vi "Get Selection from TreeBrowserWF.vi"(8 "error in (no error)":errorcluster, 10 "Input Channels":variant, 11 ".NET Refnum in":refnum<k24>) -> (0 "error out":errorcluster, 3 "Input Channel Selections":T1[](array[typedef]))   [LabVIEW 2019, in "Protection and Counter Support System Explorer.lvlib"]
uses:
  Protection and Counter Support System Explorer.lvlib
  Types/Protection Signal Linked Channel.ctl
  <vilib>/NI VeriStand/Custom Device API/Custom Device Item Ref.ctl
  NationalInstruments.VeriStand.SystemStorageUI
  NationalInstruments.VeriStand.SystemStorage
  <vilib>/NI VeriStand/Custom Device API/Custom Device API.lvlib
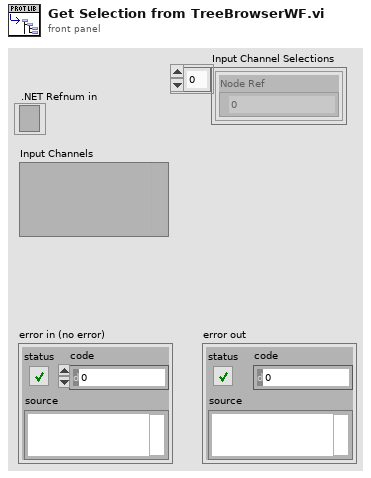
[diagram p1: front panel]
types:
  T1 = typedef "Protection and Counter Support System Explorer.lvlib/Protection Signal Linked Channel.ctl" = cluster{"Node Ref":T2}
  T2 = typedef "Custom Device API.lvlib/Custom Device Item Ref.ctl" = u64
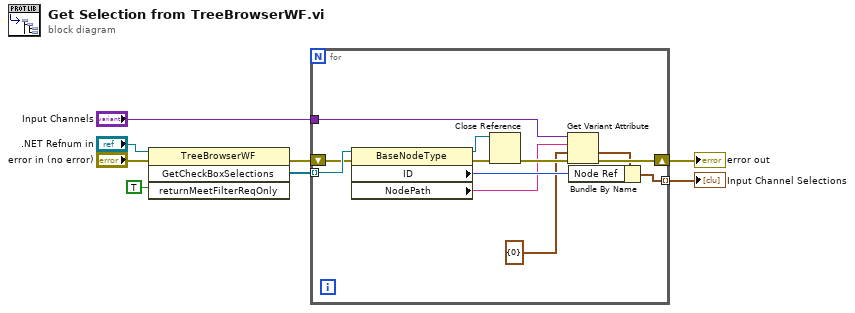
[diagram p0: block diagram]
diagram:
  n1 = invoke class="TreeBrowserWF" method="GetCheckBoxSelections"(reference=".NET Refnum in", error in="error in (no error)", "returnMeetFilterReqOnly"=TRUE) -> (error out=w5:errorcluster, "GetCheckBoxSelections"=w4:refnum<k24>[])  [unwired: 1 in, 2 out]
  n2 = for {
    tunnel: w4 -> [w20] mode=indexing
    shift-right: [w16] -> w6
    shift-left: w5 -> [w19]
    tunnel: [w17] -> w7 mode=indexing
    tunnel: "Input Channels" -> [w15]
    n3 = property class="BaseNodeType"(reference=w20, error in=w19) -> (reference out=w11:refnum<k24>, error out=w13:errorcluster, "ID"=w18:u64, "NodePath"=w10:string)
    n4 = Close Reference(reference=w11, error in (no error)=w13) -> (error out=w12:errorcluster)
    n5 = Get Variant Attribute(Variant=w15, name=w10, default value (empty Variant)=T1 {"Node Ref"=0} ("MonitoredChannelSettings"), error in=w12) -> (value=w14:T1, error out=w16:errorcluster)  [unwired: 2 out]
    n6 = Bundle By Name(cluster=w14, "Node Ref"=w18) -> (w17:T1)
  }
  "Input Channel Selections" <- w7
  "error out" <- w6
